vi "WatchdogName.vi"() -> (1 "ProcessName":string)   [LabVIEW 2017, in "GlobalConfiguration.lvlib"]
uses:
  <vilib>/addons/InsightCM/Utilities/GlobalConfiguration/GlobalConfiguration.lvlib
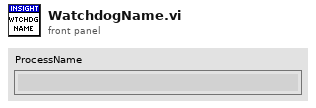
[diagram p1: front panel]
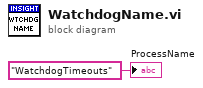
[diagram p0: block diagram]
diagram:
  "ProcessName" <- "WatchdogTimeouts" ("ProcessName")
